vi "图像格式转换不同类型.vi"() -> ()   [LabVIEW 2018]
panel:
  out "error out":errorcluster
  out "Image":T1(plugin-control)
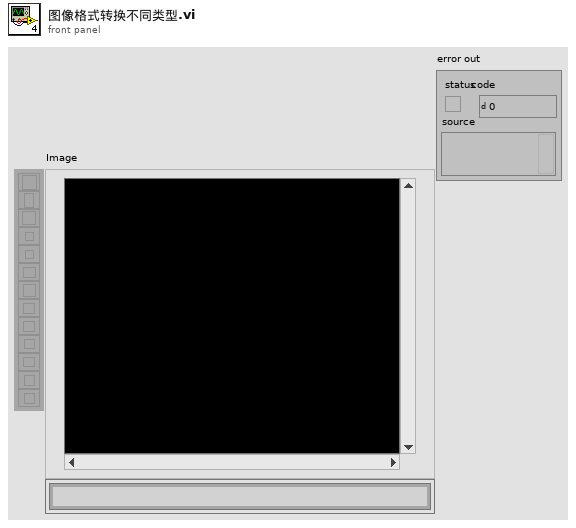
[diagram p1: front panel]
types:
  T1 = typedef "IMAQ Image.ctl" = refnum<image>
  T2 = typedef "Image Type" = u32
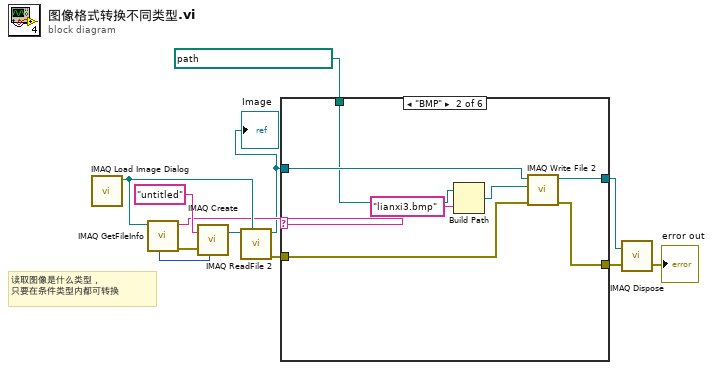
[diagram p0: block diagram]
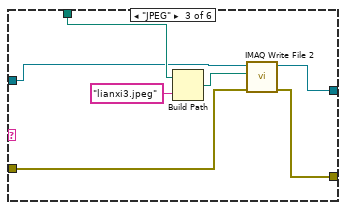
[diagram p3: hidden frame]
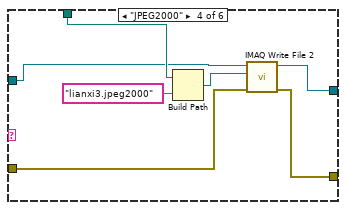
[diagram p4: hidden frame]
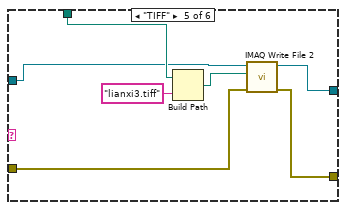
[diagram p5: hidden frame]
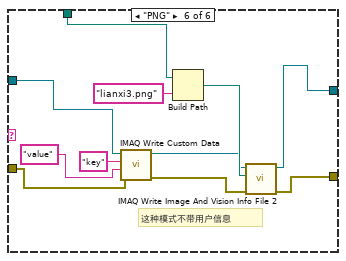
[diagram p6: hidden frame]
diagram:
  # "读取图像是什么类型，\n只要在条件类型内都可转换"
  n1 = call "IMAQ Load Image Dialog"() -> ("Path"=w9:path)  [unwired: 9 in, 2 out]
  n2 = call "IMAQ GetFileInfo"("File Path"=w9) -> ("error out"=w10:errorcluster, "File Type"=w8:string, "Image Type"=w11:T2)  [unwired: 4 in, 4 out]
  n3 = call "IMAQ Create"("Image Name"="untitled", "Image Type"=w11, "error in (no error)"=w10) -> ("New Image"=w7:T1)  [unwired: 2 in, 1 out]
  n4 = call "IMAQ ReadFile 2"("File Path"=w9, "Image"=w7) -> ("error out"=w1:errorcluster, "Image Out"=w5:T1)  [unwired: 5 in, 3 out]
  "Image" <- w5
  n5 = case shown="\"BMP\"" w8 {
    tunnel: path "D:/Labviewprogram/视觉" ("路径") -> [_ w17 w27 w34 w41 w52]
    tunnel: w5 -> [w13 w20 w25 w32 w39 w50]
    tunnel: [w13 w19 w24 w31 w38 w44] -> w4
    tunnel: [w14 w18 w23 w30 w37 w43] -> w3
    tunnel: w1 -> [w14 w15 w22 w29 w36 w51]
    frame "假", Default {
    }
    frame "BMP" {
      n6 = Build Path(base path=w17, name or relative path="lianxi3.bmp" ("名称或相对路径")) -> (appended path=w21:path)
      n7 = call-poly "IMAQ Write File 2"("error in (no error)"=w15, "File Path"=w21, "Image"=w20) -> ("error out"=w18:errorcluster, "Image Out (duplicate)"=w19:T1)  [unwired: 7 in]
    }
    frame "JPEG" {
      n8 = Build Path(base path=w27, name or relative path="lianxi3.jpeg" ("名称或相对路径")) -> (appended path=w26:path)
      n9 = call-poly "IMAQ Write File 2"("error in (no error)"=w22, "File Path"=w26, "Image"=w25) -> ("error out"=w23:errorcluster, "Image Out (duplicate)"=w24:T1)  [unwired: 7 in]
    }
    frame "JPEG2000" {
      n10 = Build Path(base path=w34, name or relative path="lianxi3.jpeg2000" ("名称或相对路径")) -> (appended path=w33:path)
      n11 = call-poly "IMAQ Write File 2"("error in (no error)"=w29, "File Path"=w33, "Image"=w32) -> ("error out"=w30:errorcluster, "Image Out (duplicate)"=w31:T1)  [unwired: 7 in]
    }
    frame "TIFF" {
      n12 = Build Path(base path=w41, name or relative path="lianxi3.tiff" ("名称或相对路径")) -> (appended path=w40:path)
      n13 = call-poly "IMAQ Write File 2"("error in (no error)"=w36, "File Path"=w40, "Image"=w39) -> ("error out"=w37:errorcluster, "Image Out (duplicate)"=w38:T1)  [unwired: 7 in]
    }
    frame "PNG" {
      # "这种模式不带用户信息"
      n14 = call "IMAQ Write Custom Data"("error in (no error)"=w51, "Custom Data In"="value", "Key"="key", "Image"=w50) -> ("error out"=w45:errorcluster, "Image Out"=w46:T1)  [unwired: 6 in]
      n15 = Build Path(base path=w52, name or relative path="lianxi3.png" ("名称或相对路径")) -> (appended path=w47:path)
      n16 = call "IMAQ Write Image And Vision Info File 2"("error in (no error)"=w45, "File Path"=w47, "Image"=w46) -> ("error out"=w43:errorcluster, "Image Out (duplicate)"=w44:T1)  [unwired: 7 in]
    }
  }
  n17 = call "IMAQ Dispose"("Image"=w4, "error in (no error)"=w3) -> ("error out"=→"error out":errorcluster)  [unwired: 4 in]
